vi "VI Server_OpenRefs.vi"(8 "error in":errorcluster, 11 "VI Path":path) -> (0 "error out":errorcluster, 3 "VI Server.RefsCluster":T1)   [LabVIEW 2020]
uses:
  VI Server_TypeDefs/VI Server_RefsCluster.ctl
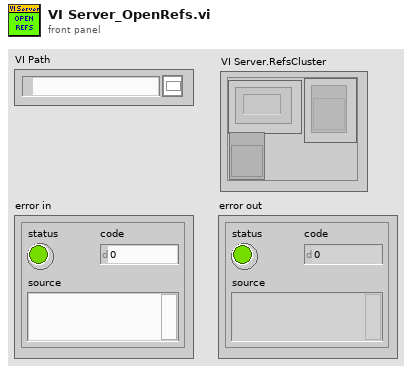
[diagram p1: front panel]
types:
  T1 = typedef "VI Server_RefsCluster.ctl" = cluster{"Labels":string[], "Refs":refnum<vi>[], "VI Ref":refnum<vi>}
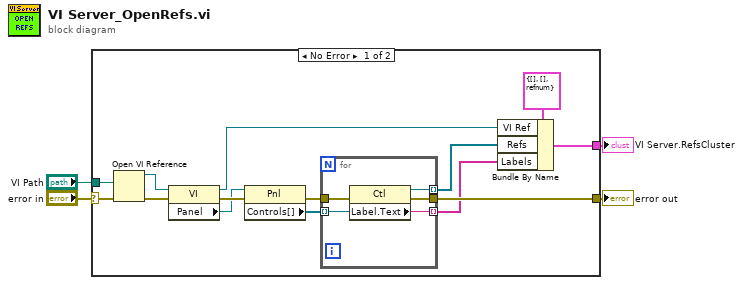
[diagram p0: block diagram]
diagram:
  n1 = case shown="No Error" "error in" {
    selector: "error in" -> [w18 w24]
    tunnel: "VI Path" -> [w16 _]
    tunnel: [w10 w24] -> w2
    tunnel: [w5 _] -> w1
    frame No Error {
      n2 = Open VI Reference(vi path=w16, error in (no error)=w18) -> (vi reference=w15:refnum<vi>, error out=w17:errorcluster)  [unwired: 4 in]
      n3 = property class="VI"(reference=w15, error in=w17) -> (reference out=w8:refnum<vi>, error out=w14:errorcluster, "Panel"=w13:refnum<vi>)
      n4 = property class="Pnl"(reference=w13, error in=w14) -> (error out=w11:errorcluster, "Controls[]"=w12:refnum<vi>[])  [unwired: 1 out]
      n5 = for {
        tunnel: w12 -> [w22] mode=indexing
        tunnel: w11 -> [w23]
        tunnel: [w21] -> w6 mode=indexing
        tunnel: [w20] -> w10
        tunnel: [w19] -> w7 mode=indexing
        n6 = property class="Ctl"(reference=w22, error in=w23) -> (reference out=w19:refnum<vi>, error out=w20:errorcluster, "Label.Text"=w21:string)
      }
      n7 = Bundle By Name(cluster=T1 {"Labels"=[], "Refs"=[], "VI Ref"=refnum} ("VI Server.RefsCluster"), "VI Ref"=w8, "Refs"=w7, "Labels"=w6) -> (w5:T1)
    }
    frame Error {
    }
  }
  "error out" <- w2
  "VI Server.RefsCluster" <- w1
